vi "RT Driver VI.vi"(7 "Operation":T9, 11 "Device Reference in":T10 format="%.0x") -> (0 "Error Code":i32)   [LabVIEW 2014, in "Waveform-Processing-Custom-Device Engine.lvlib"]
uses:
  Waveform-Processing-Custom-Device Engine.lvlib
  <vilib>/NI Veristand/Custom Device API/Custom Device Item Ref.ctl
  <vilib>/NI Veristand/Custom Device API/Hardware Interface Driver VI Operation.ctl
  Types/Inline State Vars.ctl
  Types/Async FIFOs.ctl
  Shared/CompiledSettings.ctl
  <vilib>/NI Veristand/Custom Device API/Block Data Reference.ctl
  <vilib>/NI Veristand/Custom Device API/Data Reference.ctl
  <vilib>/NI Veristand/Custom Device API/Waveform Data Reference.ctl
  Userlib/Error Handling API/Controls/Error Handling Cluster.ctl
  <vilib>/NI Veristand/Custom Device API/NI VeriStand - Set Channel Value by Data Reference.vi
  <vilib>/NI Veristand/Custom Device API/NI VeriStand - Get Channel Values by Block Data Reference.vi
  Asynchronous/Asynchronous Engine.vi
  <vilib>/NI Veristand/Custom Device API/Global Data Refs.vi
  Userlib/Inline Async API/Inline Async API.lvlib
  Userlib/Error Handling API/Error Handling API.lvlib
  <vilib>/NI Veristand/Custom Device API/Custom Device API.lvlib
  Shared/Waveform-Processing-Custom-Device Shared.lvlib
panel:
  out "Run-time State":T8 {"State Vars out"."CompiledSettings"."Result Ch Data Refs" format="%.0x"; "State Vars out"."CompiledSettings"."Parameter Block Data Refs"."Data Reference" format="%.0x"}
  out "Parameter FIFO Write Occured":bool
  out "Result FIFO Read Occured":bool
  out "Inline Loop Rate":u32
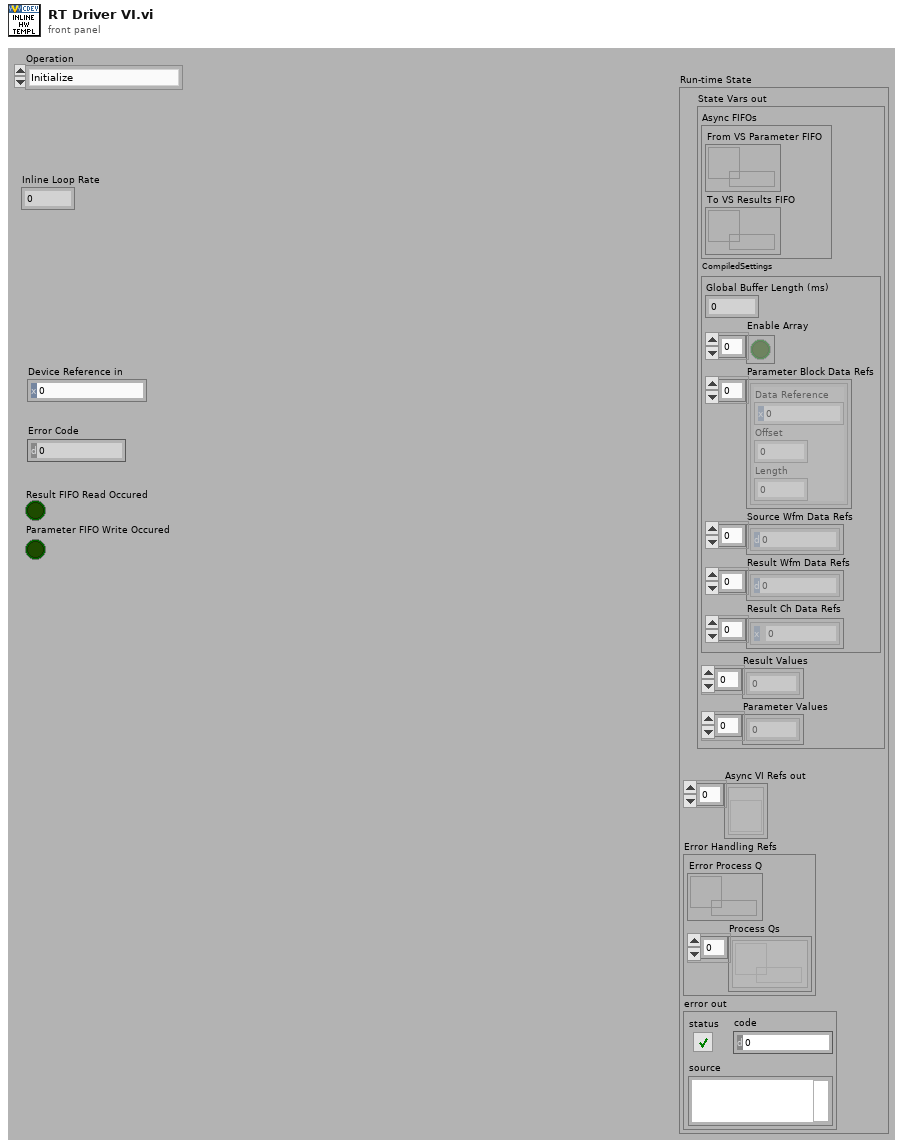
[diagram p1: front panel]
types:
  T1 = typedef "Waveform-Processing-Custom-Device Engine.lvlib/Inline State Vars.ctl" = cluster{"Async FIFOs":T2, "CompiledSettings":T3, "Result Values":dbl[], "Parameter Values":dbl[]}
  T2 = typedef "Waveform-Processing-Custom-Device Engine.lvlib/Async FIFOs.ctl" = cluster{"From VS Parameter FIFO":refnum<k33>, "To VS Results FIFO":refnum<k33>}
  T3 = typedef "Waveform-Processing-Custom-Device Shared.lvlib/CompiledSettings.ctl" = cluster{"Global Buffer Length (ms)":dbl, "Enable Array":bool[], "Parameter Block Data Refs":T4[], "Source Wfm Data Refs":T6[], "Result Wfm Data Refs":T6[], "Result Ch Data Refs":T5[]}
  T4 = typedef "Custom Device API.lvlib/Block Data Reference.ctl" = cluster{"Data Reference":T5, "Offset":i32, "Length":i32}
  T5 = typedef "Custom Device API.lvlib/Data Reference.ctl" = i32
  T6 = typedef "Custom Device API.lvlib/Waveform Data Reference.ctl" = i32
  T7 = typedef "Waveform-Processing-Custom-Device Engine.lvlib/Error Handling API.lvlib/Error Handling Cluster.ctl" = cluster{"Error Process Q":refnum<queue>, "Process Qs":refnum<queue>[]}
  T8 = cluster{"State Vars out":T1, "Async VI Refs out":refnum<vi>[], "Error Handling Refs":T7, "error out":errorcluster}
  T9 = typedef "Custom Device API.lvlib/Hardware Interface Driver VI Operation.ctl" = enum16{"Initialize", "Start", "Read Data from HW", "Write Data to HW", "Close"}
  T10 = typedef "Custom Device API.lvlib/Custom Device Item Ref.ctl" = u64
  T11 = enum32{"Invalid", "Standard", "Closed", "Hidden", "Minimized", "Maximized"}
  T12 = typedef "Waveform-Processing-Custom-Device Engine.lvlib/Async Parameters.ctl" = cluster{"Async FIFOs":T2, "Source Wfm Data Refs":T6[], "Result Wfm Data Refs":T6[], "Enable Array":bool[]}
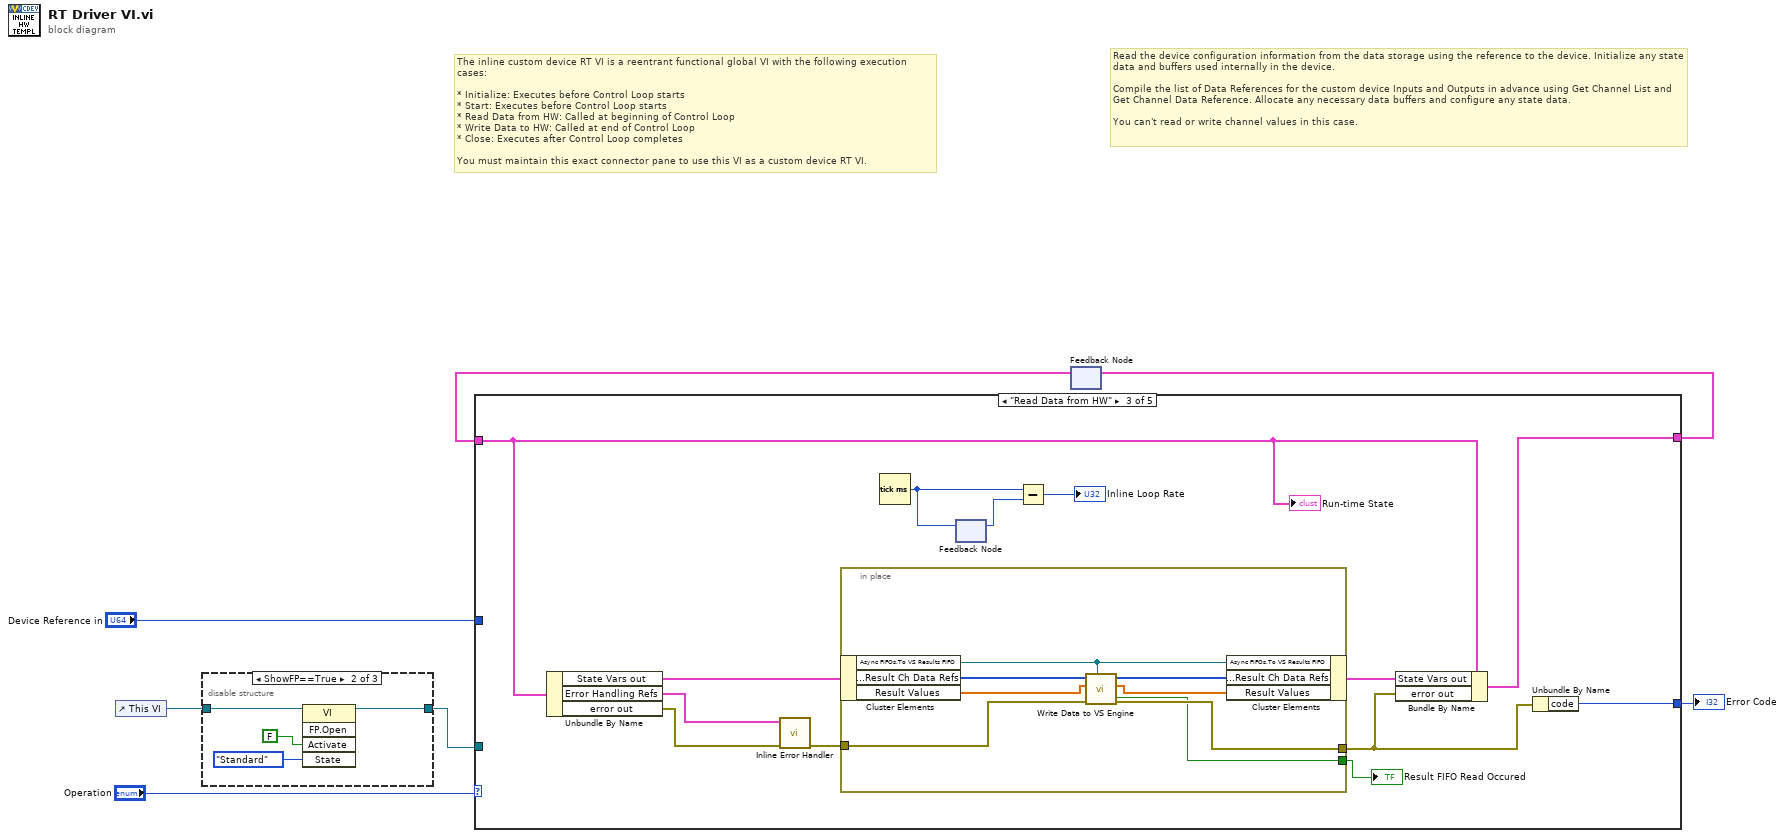
[diagram p0: block diagram]
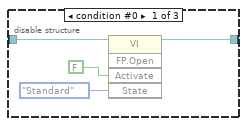
[diagram p2: hidden frame]
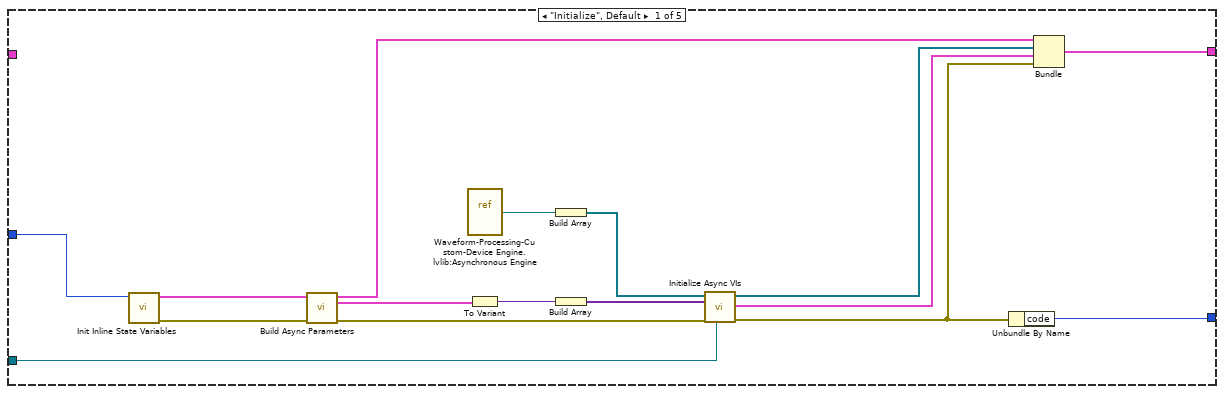
[diagram p4: hidden frame]
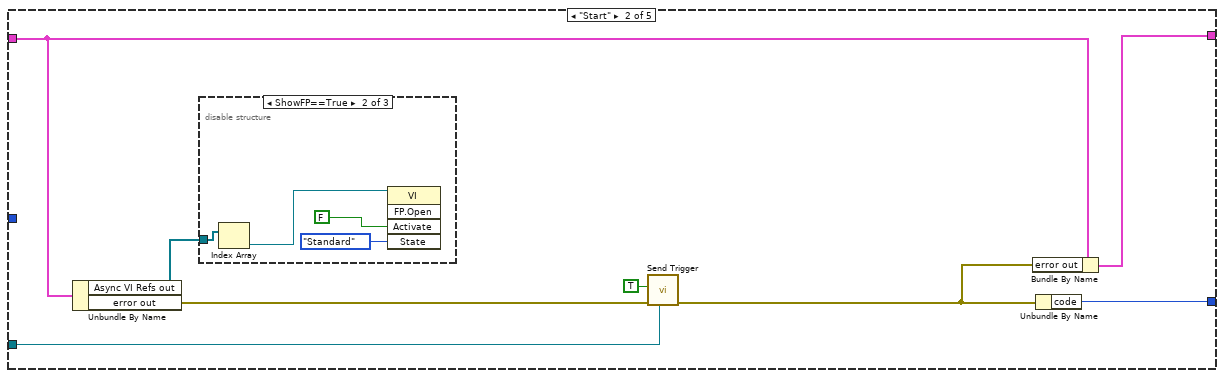
[diagram p5: hidden frame]
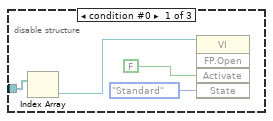
[diagram p6: hidden frame]
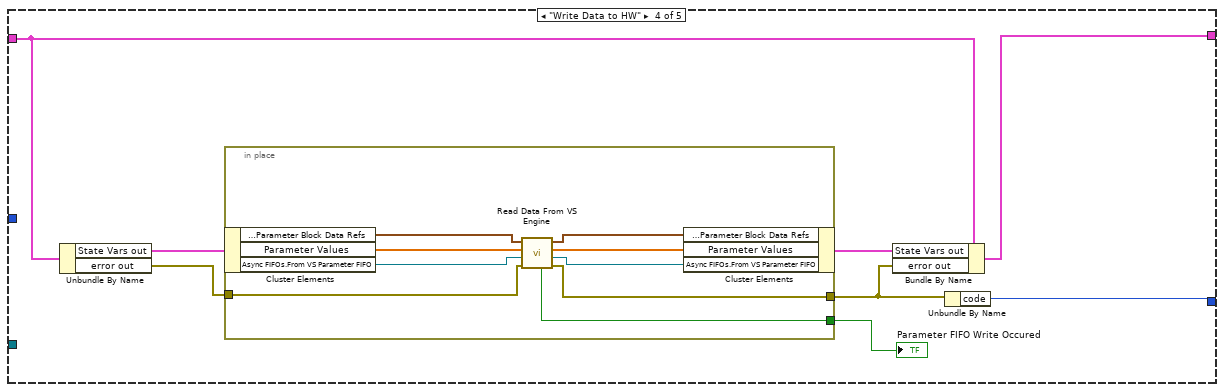
[diagram p8: hidden frame]
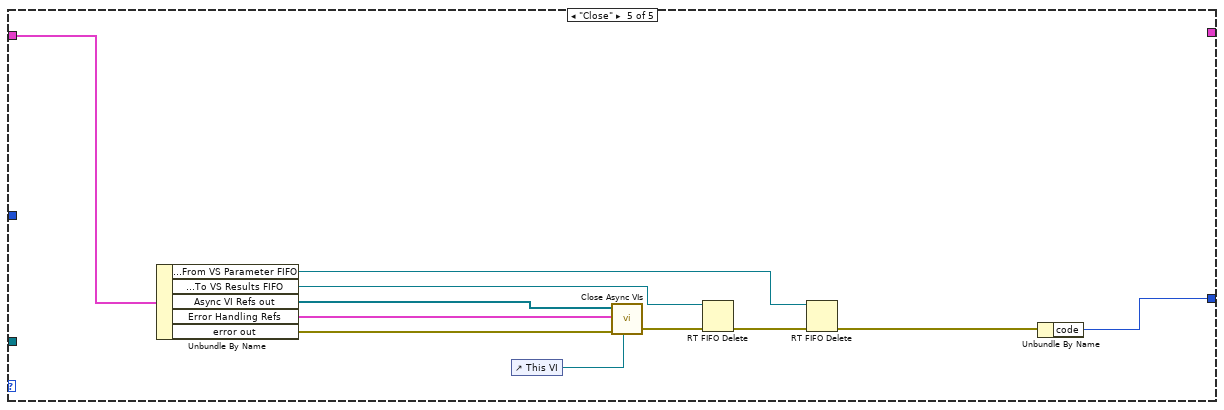
[diagram p9: hidden frame]
diagram:
  # "Read the device configuration information from the data storage using the reference to the device. Initialize any state data and buffers used internally in the device.\n\nCompile the list of Data References for the custom device Inputs and Outputs in advance using Get Channel List and Get Channel Data Reference. Allocate any necessary data buffers and configure any state data.\n\nYou can't read or write channel values in this case."
  # "The inline custom device RT VI is a reentrant functional global VI with the following execution cases:\n\n* Initialize: Executes before Control Loop starts\n* Start: Executes before Control Loop starts\n* Read Data from HW: Called at beginning of Control Loop\n* Write Data to HW: Called at end of Control Loop\n* Close: Executes after Control Loop completes\n\nYou must maintain this exact connector pane to use this VI as a custom device RT VI."
  n1 = control-ref of="This VI"() -> (w3:refnum<vi>)
  n2 = disable-structure shown="ShowFP==True" {
    disable-tunnel: w3 -> [w11 w15 w16]
    disable-tunnel: [w8 w12 w16] -> w2
    frame condition #0 {
      n3 = invoke class="VI" method="FP.Open"(reference=w11, "Activate"=FALSE ("Activate?"), "State"=T11."Standard") -> (reference out=w8:refnum<vi>)  [unwired: 2 in, 4 out]
    }
    frame condition #1 (active) {
      n4 = invoke class="VI" method="FP.Open"(reference=w15, "Activate"=FALSE ("Activate?"), "State"=T11."Standard") -> (reference out=w12:refnum<vi>)  [unwired: 2 in, 4 out]
    }
    frame condition #2 {
    }
  }
  n5 = feedback #1() -> (w6:T8)  [unwired: 1 out]
  n6 = case shown="\"Read Data from HW\"" "Operation" {
    tunnel: w6 -> [_ w36 w52 w74 w92]
    tunnel: "Device Reference in" -> [w23 _ _ _ _]
    tunnel: [w28 w39 w61 w71 w94] -> w5
    tunnel: w2 -> [w24 w33 _ _ _]
    tunnel: [w18 w34 w49 w72 _] -> w1
    frame "Initialize", Default {
      n7 = call "Init Inline State Variables.vi"("Device Reference in"=w23) -> ("error out"=w22:errorcluster, "State Vars"=w21:T1)  [unwired: 9 in]
      n8 = call "Build Async Parameters.vi"("Error in"=w22, "State Vars"=w21) -> ("Error out"=w17:errorcluster, "Async Parameters"=w19:T12, "State Vars out"=w20:T1)  [unwired: 7 in]
      n9 = vi-ref "Waveform-Processing-Custom-Device Engine.lvlib:Asynchronous Engine.vi"() -> (w32:refnum<vi>)
      n10 = To Variant(anything=w19) -> (Variant=w30:variant)
      n11 = Build Array(w32) -> (w31:refnum<vi>[])
      n12 = Build Array(w30) -> (w29:variant[])
      n13 = call "Initialize Async VIs.vi"("VI in"=w24, "error in (no error)"=w17, "Async VI Parameters"=w29, "Async VI Refs"=w31) -> ("error out"=w27:errorcluster, "Error Handling Refs"=w26:T7, "Async VI Refs out"=w25:refnum<vi>[])  [unwired: 5 in]
      n14 = Unbundle By Name(w27) -> ("code"=w28:i32)
      n15 = Bundle("State Vars out"=w20, "Async VI Refs out"=w25, "Error Handling Refs"=w26, "error out"=w27) -> (w18:T8)  [unwired: 1 in]
    }
    frame "Start" {
      n16 = Unbundle By Name(w36) -> ("Async VI Refs out"=w35:refnum<vi>[], "error out"=w37:errorcluster)
      n17 = disable-structure shown="ShowFP==True" {
        disable-tunnel: w35 -> [w42 w46 _]
        frame condition #0 {
          n18 = Index Array(array=w42) -> (element=w41:refnum<vi>)  [unwired: 1 in]
          n19 = invoke class="VI" method="FP.Open"(reference=w41, "Activate"=FALSE ("Activate?"), "State"=T11."Standard") -> ()  [unwired: 2 in, 5 out]
        }
        frame condition #1 (active) {
          n20 = Index Array(array=w46) -> (element=w45:refnum<vi>)  [unwired: 1 in]
          n21 = invoke class="VI" method="FP.Open"(reference=w45, "Activate"=FALSE ("Activate?"), "State"=T11."Standard") -> ()  [unwired: 2 in, 5 out]
        }
        frame condition #2 {
        }
      }
      n22 = call "Send Trigger.vi"("Parent VI"=w33, "error in (no error)"=w37, "notification"=TRUE) -> ("error out"=w38:errorcluster)  [unwired: 8 in]
      n23 = Bundle By Name(cluster=w36, "error out"=w38) -> (w34:T8)
      n24 = Unbundle By Name(w38) -> ("code"=w39:i32)
    }
    frame "Read Data from HW" {
      n25 = Unbundle By Name(w52) -> ("State Vars out"=w56:T1, "Error Handling Refs"=w54:T7, "error out"=w55:errorcluster)
      n26 = call "Inline Error Handler.vi"("error in"=w55, "Error Handling Cluster"=w54) -> ("error out"=w53:errorcluster)  [unwired: 9 in]
      n27 = in-place {
        in-place-border: [w69] -> w50
        in-place-border: [w68] -> w57
        in-place-border: w53 -> [w67]
        n28 = in-place-cluster #2(w56) -> ("Async FIFOs.To VS Results FIFO"=w66:refnum<k33>, "CompiledSettings.Result Ch Data Refs"=w62:T5[], "Result Values"=w65:dbl[])
        n29 = call "Write Data to VS Engine.vi"("Write to VS Engine FIFO"=w66, "error in"=w67, "Values"=w65, "Result Ch Data Refs"=w62) -> ("error out"=w69:errorcluster, "Read Occured"=w68:bool, "Values out"=w64:dbl[], "Result Ch Data Refs out"=w63:T5[])  [unwired: 4 in]
        n30 = in-place-cluster #2("Async FIFOs.To VS Results FIFO"=w66, "CompiledSettings.Result Ch Data Refs"=w63, "Result Values"=w64) -> (w51:T1)
      }
      "Result FIFO Read Occured" <- w57
      n31 = Tick Count (ms)() -> (millisecond timer value=w60:u32)
      n32 = feedback-in #3(w60) -> ()
      n33 = feedback #3() -> (w59:u32)  [unwired: 1 in]
      n34 = Subtract(x=w60, y=w59) -> (x-y=→"Inline Loop Rate":u32)
      n35 = Bundle By Name(cluster=w52, "State Vars out"=w51, "error out"=w50) -> (w49:T8)
      n36 = Unbundle By Name(w50) -> ("code"=w61:i32)
      "Run-time State" <- w52
    }
    frame "Write Data to HW" {
      n37 = Unbundle By Name(w74) -> ("State Vars out"=w77:T1, "error out"=w76:errorcluster)
      n38 = in-place {
        in-place-border: w76 -> [w86]
        in-place-border: [w81] -> w70
        in-place-border: [w80] -> w75
        n39 = in-place-cluster #4(w77) -> ("CompiledSettings.Parameter Block Data Refs"=w84:T4[], "Parameter Values"=w85:dbl[], "Async FIFOs.From VS Parameter FIFO"=w78:refnum<k33>)
        n40 = call "Read Data From VS Engine.vi"("error in"=w86, "Read from VS Engine FIFO"=w78, "Values Array"=w85, "Block Data Ref"=w84) -> ("error out"=w81:errorcluster, "Read from VS Engine FIFO out"=w79:refnum<k33>, "Values Array out"=w82:dbl[], "Block Data Ref out"=w83:T4[], "Write Occured"=w80:bool)  [unwired: 3 in]
        n41 = in-place-cluster #4("CompiledSettings.Parameter Block Data Refs"=w83, "Parameter Values"=w82, "Async FIFOs.From VS Parameter FIFO"=w79) -> (w73:T1)
      }
      "Parameter FIFO Write Occured" <- w75
      n42 = Bundle By Name(cluster=w74, "State Vars out"=w73, "error out"=w70) -> (w72:T8)
      n43 = Unbundle By Name(w70) -> ("code"=w71:i32)
    }
    frame "Close" {
      n44 = Unbundle By Name(w92) -> ("State Vars out.Async FIFOs.From VS Parameter FIFO"=w87:refnum<k33>, "State Vars out.Async FIFOs.To VS Results FIFO"=w88:refnum<k33>, "Async VI Refs out"=w89:refnum<vi>[], "Error Handling Refs"=w90:T7, "error out"=w91:errorcluster)
      n45 = control-ref of="This VI"() -> (w97:refnum<vi>)
      n46 = call "Close Async VIs.vi"("TopLevel VI"=w97, "error in (no error)"=w91, "Error Handling Refs"=w90, "Async VI"=w89) -> ("error out"=w96:errorcluster)  [unwired: 7 in]
      n47 = RT FIFO Delete(0:w88, 3:w96) -> (11:w95:errorcluster)  [unwired: 1 in]
      n48 = RT FIFO Delete(0:w87, 3:w95) -> (11:w93:errorcluster)  [unwired: 1 in]
      n49 = Unbundle By Name(w93) -> ("code"=w94:i32)
    }
  }
  "Error Code" <- w5
  n50 = feedback-in #1(w1) -> ()
